vi "Vpmt.vi"(7 "LVWS Req":refnum<class "Web Request.lvclass">, 11 "V":string) -> ()   [LabVIEW 2014]
uses:
  <vilib>/wsapi/Web Request.lvclass
  Instr Actor/Messages/Update PMT Gains MSG/Update PMT Gains MSG.lvclass
  Controller/Controls/Enqueuer Enum.ctl
  Instr Actor/Messages/Update PMT Gains MSG/Update PMT Gains MSG.lvclass/Update PMT Gains MSG.ctl
  Controller/Controller.lvclass
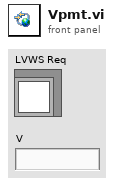
[diagram p1: front panel]
types:
  T1 = typedef "Controller.lvlib/Controller.lvclass/Enqueuer Enum.ctl" = enum8{"PAS", "CRDS", "File", "O3Lamp"}
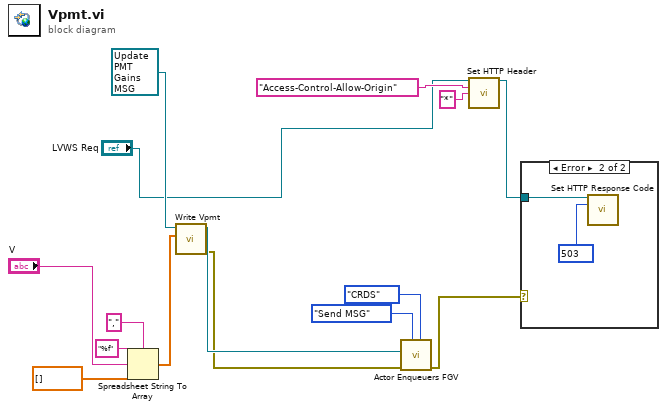
[diagram p0: block diagram]
diagram:
  n1 = Spreadsheet String To Array(delimiter (Tab)=",", format string="%f", spreadsheet string="V", array type (2D Dbl)=dbl[] []) -> (array=w9:dbl[])
  n2 = call "Write Vpmt.vi"("Vpmt"=w9, "Update PMT Gains MSG in"=refnum<class "Update PMT Gains MSG.lvclass"> refnum ("Instrument Lib:Update PMT Gains MSG.lvclass")) -> ("error out"=w5:errorcluster, "Update PMT Gains MSG out"=w8:refnum<class "Update PMT Gains MSG.lvclass">)  [unwired: 8 in]
  n3 = call "Actor Enqueuers FGV.vi"("Enqueuer"=Enqueuer_Enum."CRDS", "State"=enum16{"Store", "Send MSG"}."Send MSG", "error in"=w5, "MSG"=w8) -> ("error out"=w11:errorcluster)  [unwired: 7 in]
  n4 = call <vilib>:"Set HTTP Header.vi"("LabVIEW Web Service Request"="LVWS Req", "header"="Access-Control-Allow-Origin", "header value"="*") -> ("LabVIEW Web Service Request out"=w1:refnum<class "Web Request.lvclass">)  [unwired: 11 in, 1 out]
  n5 = case shown="Error" w11 {
    tunnel: w1 -> [_ w17]
    frame No Error {
    }
    frame Error {
      w16 = 503 items=["100"=100, "101"=101, "200"=200, "201"=201, "202"=202, "203"=203, "204"=204, "205"=205, "206"=206, "300"=300, "301"=301, "302"=302, "303"=303, "304"=304, "305"=305, "306"=306, "307"=307, "400"=400, "401"=401, "402"=402, "403"=403, "404"=404, "405"=405, "406"=406, "407"=407, "408"=408, "409"=409, "410"=410, "411"=411, "412"=412, "413"=413, "414"=414, "415"=415, "416"=416, "417"=417, "500"=500, "501"=501, "502"=502, "503"=503, "504"=504, "505"=505] ("response code (200)")
      n6 = call <vilib>:"Set HTTP Response Code.vi"("LabVIEW Web Service Request"=w17, "response code (200)"=w16) -> ()  [unwired: 12 in, 2 out]
    }
  }
